vi "EndExperiment.vi"(8 "error in (no error)":errorcluster, 11 "TrialBasedExperiment in":refnum<class "MatlabExperiment.lvclass">) -> (0 "error out":errorcluster, 3 "TrialBasedExperiment out":refnum<class "MatlabExperiment.lvclass">)   [LabVIEW 2014, in "AcquisitionCoreObjects.lvlib" / "MatlabExperiment.lvclass"]
uses:
  MatlabExperiment.lvclass
  TrialBasedExperimentObject/TrialBasedExperiment.lvclass
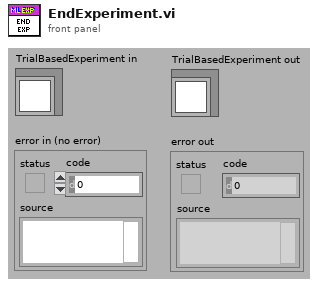
[diagram p1: front panel]
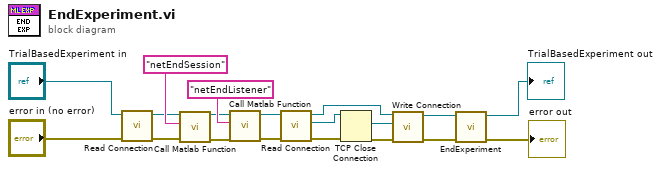
[diagram p0: block diagram]
diagram:
  n1 = call-dynamic "Read Connection.vi"("error in (no error)"="error in (no error)", "TrialBasedExperiment in"="TrialBasedExperiment in") -> ("error out"=w7:errorcluster, "TrialBasedExperiment out"=w9:refnum<class "MatlabExperiment.lvclass">)  [unwired: 7 in, 1 out]
  n2 = call-dynamic "Call Matlab Function.vi"("error in (no error)"=w7, "Function name"="netEndSession", "TrialBasedExperiment in"=w9) -> ("error out"=w6:errorcluster, "TrialBasedExperiment out"=w14:refnum<class "MatlabExperiment.lvclass">)  [unwired: 5 in, 2 out]
  n3 = call-dynamic "Call Matlab Function.vi"("error in (no error)"=w6, "Function name"="netEndListener", "TrialBasedExperiment in"=w14) -> ("error out"=w5:errorcluster, "TrialBasedExperiment out"=w13:refnum<class "MatlabExperiment.lvclass">)  [unwired: 5 in, 2 out]
  n4 = call-dynamic "Read Connection.vi"("error in (no error)"=w5, "TrialBasedExperiment in"=w13) -> ("error out"=w11:errorcluster, "Connection"=w12:refnum<k5>, "TrialBasedExperiment out"=w8:refnum<class "MatlabExperiment.lvclass">)  [unwired: 7 in]
  n5 = TCP Close Connection(connection ID=w12, error in (no error)=w11) -> (connection ID out=w10:refnum<k5>, error out=w17:errorcluster)  [unwired: 1 out]
  n6 = call-dynamic "Write Connection.vi"("error in (no error)"=w17, "Connection"=w10, "TrialBasedExperiment in"=w8) -> ("error out"=w3:errorcluster, "TrialBasedExperiment out"=w4:refnum<class "MatlabExperiment.lvclass">)  [unwired: 7 in]
  n7 = call-parent "EndExperiment.vi"("error in (no error)"=w3, "TrialBasedExperiment in"=w4) -> ("error out"=→"error out":errorcluster, "TrialBasedExperiment out"=→"TrialBasedExperiment out":refnum<class "MatlabExperiment.lvclass">)  [unwired: 8 in]
